vi "Adjust Input Range.vi"(8 "error in":errorcluster, 10 "Range Input":cluster{"high":dbl, "low":dbl}, 11 "Humidity Control in":refnum<class "Humidity Control.lvclass">) -> (0 "error out":errorcluster, 3 "Humidity Control out":refnum<class "Humidity Control.lvclass">)   [LabVIEW 2012]
doc: "Adjust the input control range for the control loop. This VI is generally used to set bounds on the PID output range."
uses:
  Humidity Control.lvclass
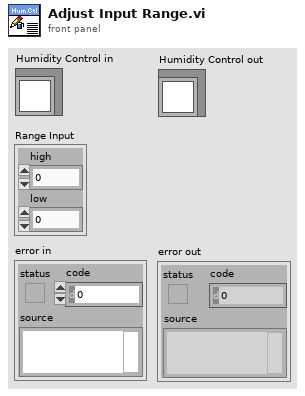
[diagram p1: front panel]
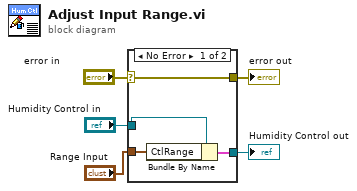
[diagram p0: block diagram]
diagram:
  n1 = case shown="No Error" "error in" {
    selector: "error in" -> [w9 w11]
    tunnel: [w9 w11] -> w4
    tunnel: [w6 w10] -> w2
    tunnel: "Humidity Control in" -> [w8 w10]
    tunnel: "Range Input" -> [w7 _]
    frame No Error {
      n2 = Bundle By Name(cluster=w8, "CtlRange"=w7) -> (w6:cluster{})
    }
    frame Error {
    }
  }
  "error out" <- w4
  "Humidity Control out" <- w2
